vi "Configure Laser AI.vi"(8 "error in":errorcluster, 11 "cCRDS in":refnum<class "cCRDS.lvclass">=refnum) -> (0 "error out":errorcluster, 1 "dt":dbl, 3 "cCRDS out":refnum<class "cCRDS.lvclass">)   [LabVIEW 2015, in "cCRDS.lvclass"]
uses:
  cCRDS.lvclass
  cCRDS.lvclass/cCRDS.ctl
  <vilib>/DAQmx/configure/timing.llb/DAQmx Timing (Implicit).vi
  <vilib>/DAQmx/configure/timing.llb/DAQmx Timing (Sample Clock).vi
  Data Access/Write Gate CO.vi
  Data Access/Write AI.vi
  <resource>/objmgr/daqmx.rc
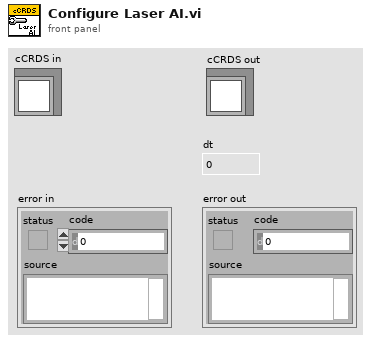
[diagram p1: front panel]
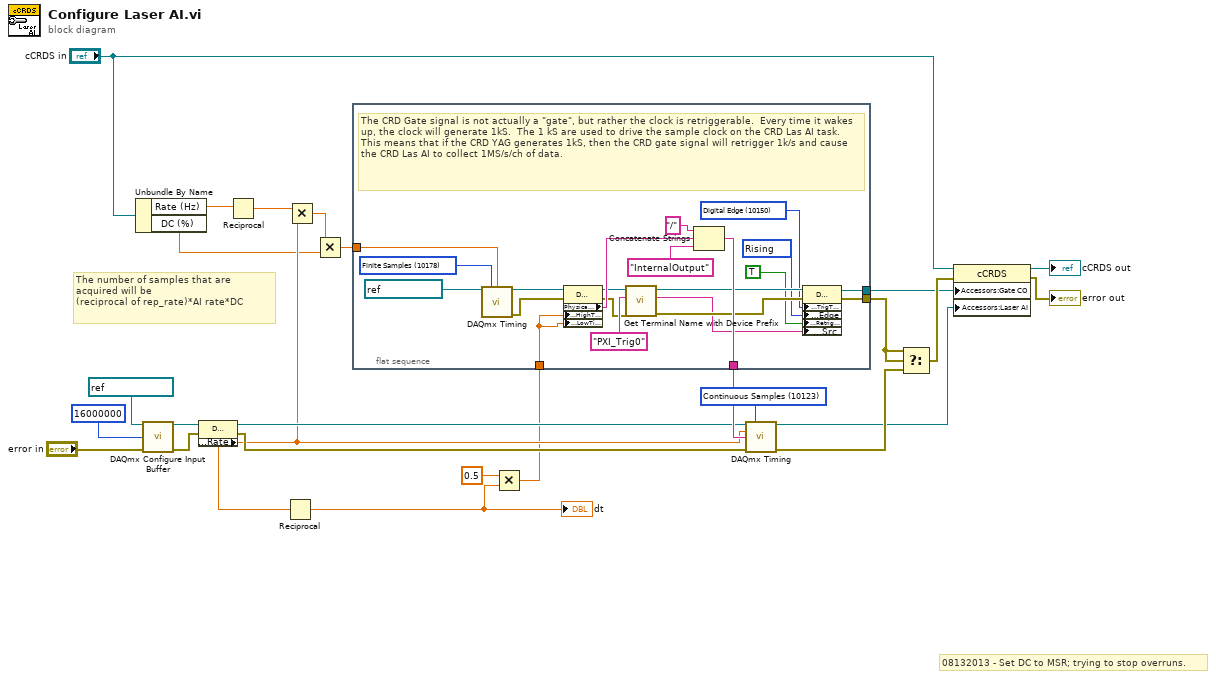
[diagram p0: block diagram]
diagram:
  w21 = 10123 items=["Finite Samples"=10178, "Continuous Samples"=10123, "Hardware Timed Single Point"=12522] ("sample mode")
  # "The number of samples that are acquired will be\n(reciprocal of rep_rate)*AI rate*DC"
  # "08132013 - Set DC to MSR; trying to stop overruns."
  n1 = Unbundle By Name("cCRDS in") -> ("Rate (Hz)"=w11:sgl, "DC (%)"=w6:sgl)
  n2 = call <vilib>:"DAQmx Configure Input Buffer.vi"("task/channels in"=refnum<k21> "CRD Las AI" ("Laser AI"), "buffer size (in samples per channel)"=u32 16000000, "error in"="error in") -> ("task out"=w16:refnum<k21>, "error out"=w14:errorcluster)  [unwired: 11 in]
  n3 = property class="DAQmx Timing"(reference=w16, error in=w14) -> (reference out=w19:refnum<k21>, error out=w18:errorcluster, "SampClk.Rate"=w9:dbl)
  n4 = Reciprocal(x=w11) -> (1/x=w10:sgl)
  n5 = Reciprocal(x=w9) -> (1/x=w5:dbl)
  "dt" <- w5
  n6 = Multiply(x=w10, y=w9) -> (x*y=w8:dbl)
  n7 = Multiply(x=w8, y=w6) -> (x*y=w7:dbl)
  n8 = flat-sequence {
    tunnel: [w47] -> w25
    tunnel: [w36] -> w22
    tunnel: [w35] -> w20
    tunnel: w7 -> [w28]
    tunnel: w3 -> [w27]
    frame #0 {
      w29 = 10150 items=["Analog Edge"=10099, "Digital Edge"=10150, "Digital Pattern"=10398, "Analog Window"=10103, "None"=10230] ("Start.TrigType")
      w30 = 10280 items=["Rising"=10280, "Falling"=10171] ("edge")
      w45 = 10178 items=["Finite Samples"=10178, "Continuous Samples"=10123, "Hardware Timed Single Point"=12522] ("sample mode")
      # "The CRD Gate signal is not actually a \"gate\", but rather the clock is retriggerable.  Every time it wakes up, the clock will generate 1kS.  The 1 kS are used to drive the sample clock on the CRD Las AI task.  This means that if the CRD YAG generates 1kS, then the CRD gate signal will retrigger 1k/s and cause the CRD Las AI to collect 1MS/s/ch of data."
      n9 = call-poly <vilib>:"DAQmx Timing.vi"("task/channels in"=refnum<k21> "CRD Gate" ("Laser AI"), "sample mode"=w45, "samples per channel"=w28) -> ("task out"=w44:refnum<k21>, "error out"=w43:errorcluster)  [unwired: 1 in, 10 out]
      n10 = property class="DAQmx Channel"(reference=w44, error in=w43, "CO.Pulse.HighTime"=w27, "CO.Pulse.LowTime"=w27) -> (reference out=w39:refnum<k21>, error out=w37:errorcluster, "PhysicalChanName"=w40:tag)
      n11 = call "Get Terminal Name with Device Prefix.vi"("error in"=w37, "Local Terminal Name"="PXI_Trig0", "task/channels in"=w39) -> ("error out"=w33:errorcluster, "Terminal Name with Device Prefix"=w31:tag, "task out"=w34:refnum<k21>)  [unwired: 6 in]
      n12 = Concatenate Strings("/", w40, "InternalOutput" ("string")) -> (w36:string)
      n13 = property class="DAQmx Trigger"(reference=w34, error in=w33, "Start.TrigType"=w29, "Start.DigEdge.Edge"=w30, "Start.Retriggerable"=TRUE, "Start.DigEdge.Src"=w31) -> (reference out=w47:refnum<k21>, error out=w35:errorcluster)
    }
  }
  n14 = Multiply(x=0.5, y=w5) -> (x*y=w3:dbl)
  n15 = call-poly <vilib>:"DAQmx Timing.vi"("task/channels in"=w19, "sample mode"=w21, "rate"=w9, "source"=w22, "error in"=w18) -> ("task out"=w1:refnum<k21>, "error out"=w2:errorcluster)  [unwired: 2 in, 7 out]
  n16 = Select(t=w20, s=w20, f=w2) -> (s? t:f=w26:errorcluster)
  n17 = property class="cCRDS"(reference="cCRDS in", error in=w26, "Accessors:Gate CO"=w25, "Accessors:Laser AI"=w1) -> (reference out=→"cCRDS out":refnum<class "cCRDS.lvclass">, error out=→"error out":errorcluster)
